vi "set shared data ref.vi"(8 "error in (no error)":errorcluster, 10 "shared data ref":T1, 11 "Node Ptr":T2 format="%.0x") -> (0 "error out":errorcluster, 3 "Item Ref out":T2 format="%.0x")   [LabVIEW 2017, in "DSF System Explorer.lvlib"]
uses:
  DSF System Explorer.lvlib
  <vilib>/NI Veristand/Custom Device API/Custom Device Item Ref.ctl
  shared data ref.ctl
  shared data.ctl
  DSF Core.lvlibp/Classes/Configuration/Configuration Session.lvclass
  Shared/DSF Shared.lvlib
  <vilib>/NI Veristand/Custom Device API/Custom Device API.lvlib
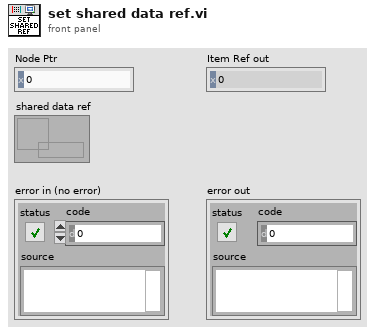
[diagram p1: front panel]
types:
  T1 = typedef "DSF System Explorer.lvlib/shared data ref.ctl" = refnum<data-value>
  T2 = typedef "Custom Device API.lvlib/Custom Device Item Ref.ctl" = u64
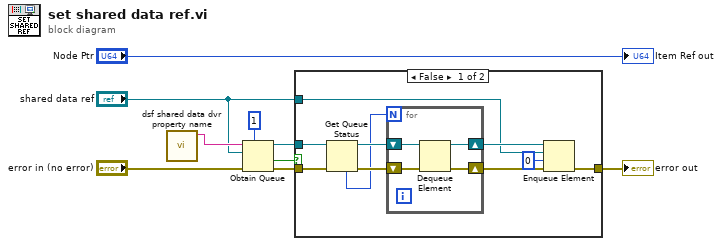
[diagram p0: block diagram]
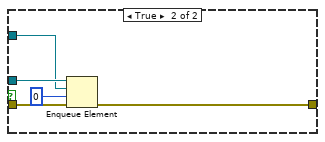
[diagram p2: hidden frame]
diagram:
  n1 = call "dsf shared data dvr property name.vi"() -> ("shared data dvr property name"=w4:string)  [unwired: 11 in]
  n2 = Obtain Queue(max queue size (-1, unlimited)=1, name (unnamed)=w4, element data type="shared data ref", error in (no error)="error in (no error)") -> (queue out=w7:refnum<queue>, created new?=w2:bool, error out=w8:errorcluster)  [unwired: 1 in]
  n3 = case shown="False" w2 {
    tunnel: w8 -> [w18 w28]
    tunnel: w7 -> [w19 w27]
    tunnel: "shared data ref" -> [w12 w26]
    tunnel: [w13 w25] -> w5
    frame False {
      n4 = Get Queue Status(queue=w19, error in (no error)=w18) -> (queue out=w16:refnum<queue>, error out=w17:errorcluster, # elements in queue=w11:i32)  [unwired: 1 in, 5 out]
      n5 = for {
        N: w11 -> [_]
        shift-right: [w20] -> w14
        shift-left: w17 -> [w22]
        shift-right: [w21] -> w15
        shift-left: w16 -> [w23]
        n6 = Dequeue Element(queue=w23, error in (no error)=w22) -> (queue out=w21:refnum<queue>, error out=w20:errorcluster)  [unwired: 1 in, 2 out]
      }
      n7 = Enqueue Element(queue=w15, element=w12, timeout in ms (-1)=0, error in (no error)=w14) -> (error out=w13:errorcluster)  [unwired: 2 out]
    }
    frame True {
      n8 = Enqueue Element(queue=w27, element=w26, timeout in ms (-1)=0, error in (no error)=w28) -> (error out=w25:errorcluster)  [unwired: 2 out]
    }
  }
  "error out" <- w5
  "Item Ref out" <- "Node Ptr"
